vi "test Acyclic Loopback with SDI.vi"(8 "error in":errorcluster, 11 "TestCase in":refnum<class "Octal Loopback.lvclass">) -> (0 "error out":errorcluster, 3 "TestCase out":refnum<class "Octal Loopback.lvclass">)   [LabVIEW 2020, in "Octal Loopback.lvclass"]
uses:
  Octal Loopback.lvclass
  C:/Program Files (x86)/National Instruments/LabVIEW 2020/vi.lib/NI/VeriStand Custom Device Testing Tools/VeriStandTestCase/VeriStandTestCase.lvclass
  <vilib>/numeric/Random Number (Range) U64.vi
  <vilib>/numeric/sub_Random U32.vi
  <vilib>/NI VeriStand/Execution/Workspace/NI VeriStand - Set Single Channel Value.vi
  <vilib>/addons/_JKI Toolkits/VI Tester/TestCase.llb/TestCase.lvclass
  <vilib>/NI VeriStand/Execution/Workspace/NI_VS Workspace ExecutionAPI.lvlib
  <vilib>/NI/VeriStand Custom Device Testing Tools/VeriStandTestUtilities/VeriStandTestUtilities.lvlib
  C:/Program Files (x86)/National Instruments/LabVIEW 2020/vi.lib/addons/_JKI Toolkits/VI Tester/TestCase.llb/TestCase.lvclass
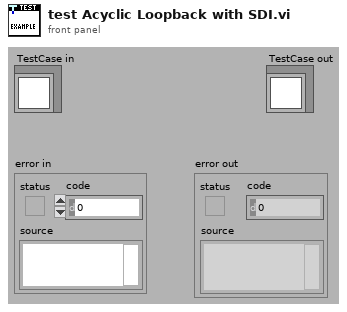
[diagram p1: front panel]
types:
  T1 = typedef "NI_VS Workspace ExecutionAPI.lvlib/WorkspaceAPI.ctl" = refnum<k24>
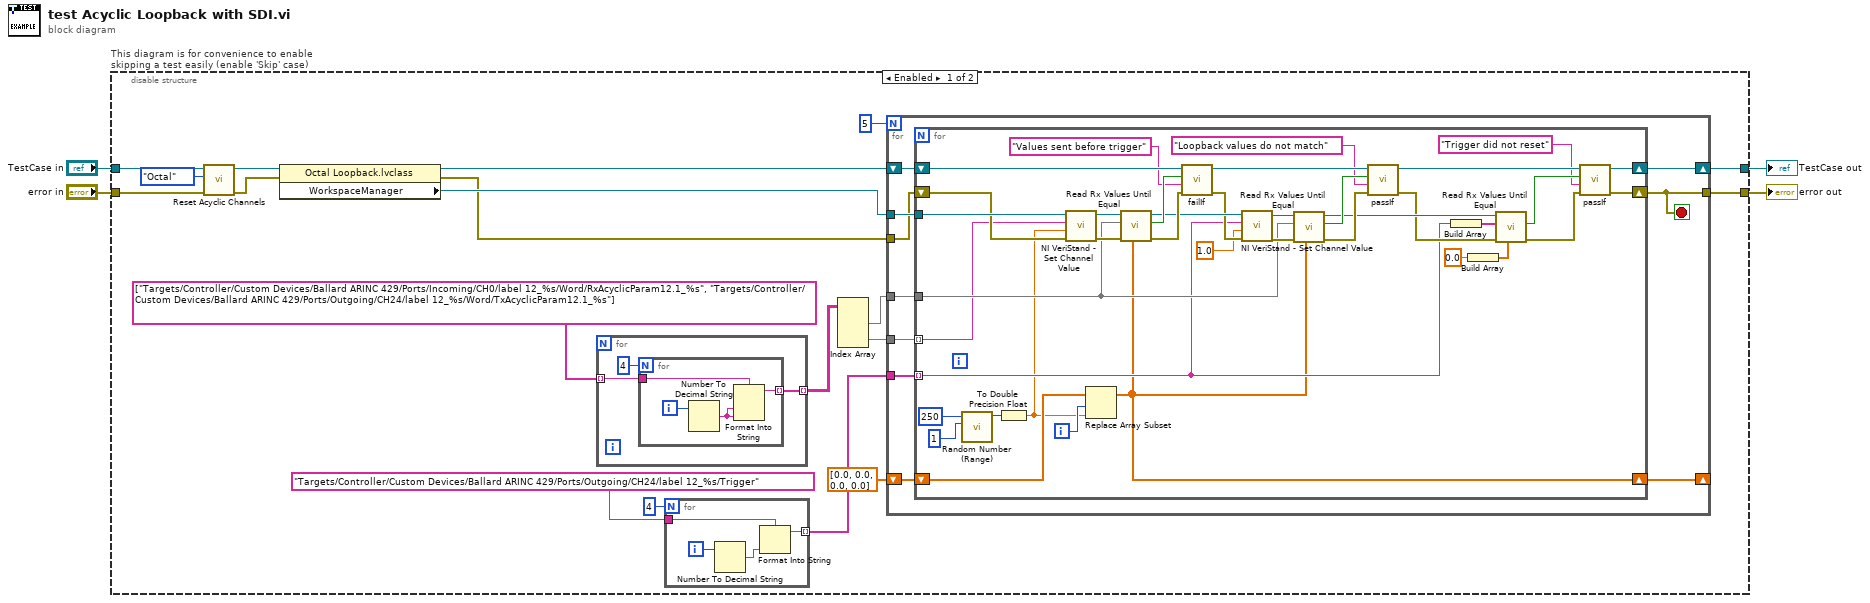
[diagram p0: block diagram]
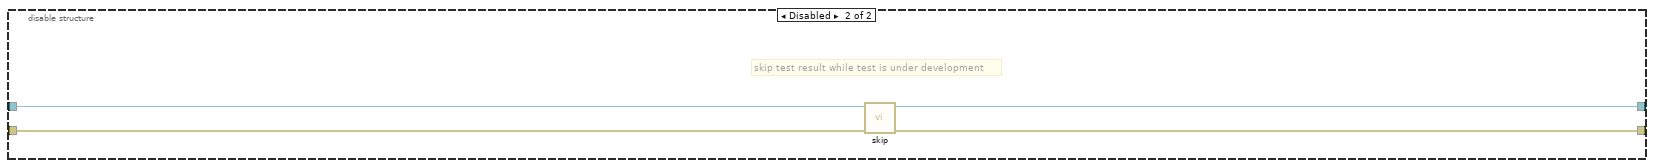
[diagram p2: hidden frame]
diagram:
  n1 = disable-structure "This diagram is for convenience to enable skipping a test easily (enable 'Skip' case)" shown="Enabled" {
    disable-tunnel: "TestCase in" -> [w15 w86]
    disable-tunnel: [w18 w84] -> w1
    disable-tunnel: [w17 w85] -> w3
    disable-tunnel: "error in" -> [w19 w83]
    frame Enabled {
      n2 = call "Reset Acyclic Channels.vi"("error in (no error)"=w19, "Label Format (Decimal)"=enum16{"Decimal", "Octal"}."Octal", "reference in"=w15) -> ("error out"=w16:errorcluster, "reference out"=w14:refnum<class "Octal Loopback.lvclass">)  [unwired: 7 in]
      n3 = property class="Octal Loopback.lvclass"(reference=w14, error in=w16) -> (reference out=w21:refnum<class "Octal Loopback.lvclass">, error out=w22:errorcluster, "WorkspaceManager"=w23:T1)
      n4 = for {
        tunnel: [w30] -> w10 mode=indexing
        tunnel: string[] ["Targets/Controller/Custom Devices/Ballard ARINC 429/Ports/Incoming/CH0/label 12_%s/Word/RxAcyclicParam12.1_%s", "Targets/Controller/Custom Devices/Ballard ARINC 429/Ports/Outgoing/CH24/label 12_%s/Word/TxAcyclicParam12.1_%s"] -> [w29] mode=indexing
        n5 = for {
          N: 4 -> [_]
          tunnel: w29 -> [w31]
          tunnel: [w33] -> w30 mode=indexing
          i -> [w34]
          n6 = Number To Decimal String(number=w34) -> (decimal integer string=w32:string)  [unwired: 1 in]
          n7 = Format Into String(format string=w31, w32, w32) -> (resulting string=w33:string)  [unwired: 2 in, 1 out]
        }
      }
      n8 = for {
        N: 4 -> [_]
        tunnel: [w26] -> w7 mode=indexing
        tunnel: "Targets/Controller/Custom Devices/Ballard ARINC 429/Ports/Outgoing/CH24/label 12_%s/Trigger" -> [w24]
        i -> [w27]
        n9 = Number To Decimal String(number=w27) -> (decimal integer string=w25:string)  [unwired: 1 in]
        n10 = Format Into String(format string=w24, w25) -> (resulting string=w26:string)  [unwired: 2 in, 1 out]
      }
      n11 = Index Array(array=w10) -> (element #1=w12:string[], element #2=w11:string[])  [unwired: 4 in]
      n12 = for {
        N: 5 -> [_]
        tunnel: w23 -> [w44]
        tunnel: w22 -> [w42]
        shift-right: [w40] -> w18
        shift-left: w21 -> [w43]
        tunnel: [w41] -> w17
        tunnel: w11 -> [w39]
        tunnel: w7 -> [w38]
        tunnel: w12 -> [w37]
        shift-right: [w36] -> _
        shift-left: dbl[] [0.0, 0.0, 0.0, 0.0] -> [w35]
        stop <- w41 stop-if-true
        n13 = for {
          tunnel: w44 -> [w81]
          shift-right: [w65] -> w40
          shift-left: w43 -> [w77]
          shift-right: [w67] -> w41
          shift-left: w42 -> [w75]
          tunnel: w39 -> [w53] mode=indexing
          tunnel: w38 -> [w52] mode=indexing
          tunnel: w37 -> [w54]
          shift-right: [w47] -> w36
          shift-left: w35 -> [w48]
          i -> [w46]
          n14 = call-poly <vilib>:"Random Number (Range).vi"("lower bound (0)"=u64 1 ("upper bound (100)"), "upper bound (100)"=u64 250) -> ("number"=w57:u64)  [unwired: 9 in]
          n15 = To Double Precision Float(number=w57) -> (double precision float=w45:dbl)
          n16 = call-poly <vilib>:"NI VeriStand - Set Channel Value.vi"("error in (no error)"=w75, "Value"=w45, "Channel"=w53, "WorkspaceManager in"=w81) -> ("error out"=w78:errorcluster, "WorkspaceManager out"=w80:T1)  [unwired: 6 in]
          n17 = Replace Array Subset(array=w48, new element=w45, index=w46) -> (w47:dbl[])
          n18 = call <vilib>:"Read Rx Values Until Equal.vi"("expected values"=w47, "error in"=w78, "Rx aliases"=w54, "workspace manager in"=w80) -> ("error out"=w79:errorcluster, "values equal expected"=w76:bool, "workspace manager out"=w74:T1)  [unwired: 5 in]
          n19 = call-dynamic "failIf.vi"("error in (no error)"=w79, "message (\"\")"="Values sent before trigger" ("message (\"\")"), "fail"=w76, "TestCase in"=w77) -> ("error out"=w73:errorcluster, "TestCase out"=w68:refnum<class "Octal Loopback.lvclass">)  [unwired: 6 in]
          n20 = call-poly <vilib>:"NI VeriStand - Set Channel Value.vi"("error in (no error)"=w73, "Value"=1.0, "Channel"=w52, "WorkspaceManager in"=w74) -> ("error out"=w71:errorcluster, "WorkspaceManager out"=w72:T1)  [unwired: 6 in]
          n21 = call <vilib>:"Read Rx Values Until Equal.vi"("expected values"=w47, "error in"=w71, "Rx aliases"=w54, "workspace manager in"=w72) -> ("error out"=w69:errorcluster, "values equal expected"=w70:bool, "workspace manager out"=w63:T1)  [unwired: 5 in]
          n22 = call-dynamic "passIf.vi"("error in (no error)"=w69, "message (\"\")"="Loopback values do not match" ("message (\"\")"), "pass"=w70, "TestCase in"=w68) -> ("error out"=w62:errorcluster, "TestCase out"=w66:refnum<class "Octal Loopback.lvclass">)  [unwired: 6 in]
          n23 = Build Array(w52) -> (w51:string[])
          n24 = Build Array(0.0) -> (w49:dbl[])
          n25 = call <vilib>:"Read Rx Values Until Equal.vi"("expected values"=w49, "error in"=w62, "Rx aliases"=w51, "workspace manager in"=w63) -> ("error out"=w61:errorcluster, "values equal expected"=w64:bool)  [unwired: 5 in, 1 out]
          n26 = call-dynamic "passIf.vi"("error in (no error)"=w61, "message (\"\")"="Trigger did not reset" ("message (\"\")"), "pass"=w64, "TestCase in"=w66) -> ("error out"=w67:errorcluster, "TestCase out"=w65:refnum<class "Octal Loopback.lvclass">)  [unwired: 6 in]
        }
      }
    }
    frame Disabled {
      # "skip test result while test is under development"
      n27 = call <vilib>:"skip.vi"("error in (no error)"=w83, "TestCase in"=w86) -> ("error out"=w85:errorcluster, "TestCase out"=w84:refnum<class "Octal Loopback.lvclass">)  [unwired: 8 in]
    }
  }
  "error out" <- w3
  "TestCase out" <- w1
